vi "Configure Instrument.vi"(0 "RFmx Handle In":refnum<k21>, 1 "Selector String":string, 7 "LO Configuration":T1 {"LO Offset Mode" items=["NoOffset", "Automatic", "User Defined"]; "LO Sharing Mode" items=["None", "Automatic", "Manual"]}, 11 "error in (no error)":errorcluster) -> (4 "RFmx Handle Out":refnum<k21>, 15 "error out":errorcluster)   [LabVIEW 2016, in "RFmxInstr.lvlib"]
uses:
  RFmxInstr.lvlib
  Typedefs/LO Configuration.ctl
  <resource>/objmgr/RFmxInstr.rc
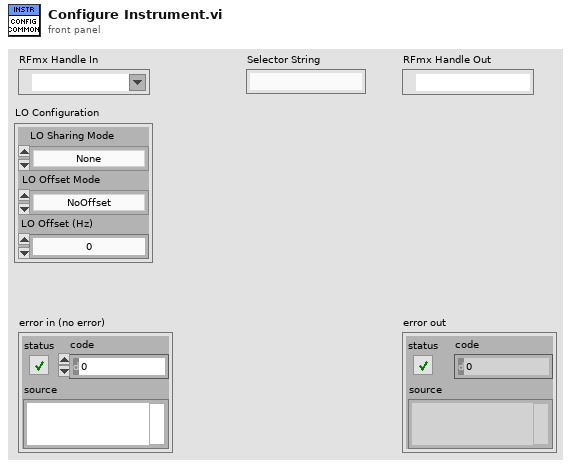
[diagram p1: front panel]
types:
  T1 = typedef "RFmxInstr.lvlib/LO Configuration.ctl" = cluster{"LO Sharing Mode":i32, "LO Offset Mode":i32, "LO Offset (Hz)":dbl}
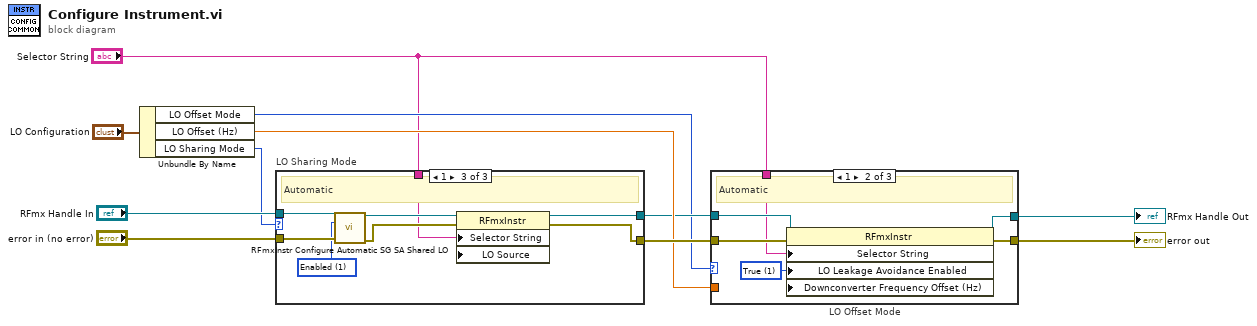
[diagram p0: block diagram]
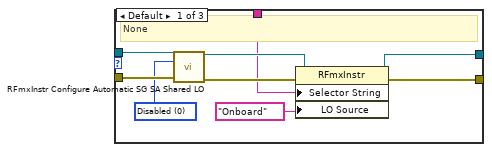
[diagram p2: hidden frame]
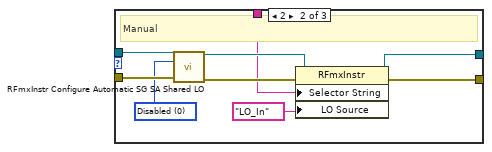
[diagram p3: hidden frame]
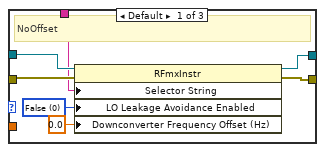
[diagram p4: hidden frame]
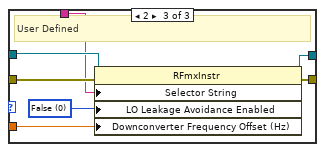
[diagram p5: hidden frame]
diagram:
  n1 = Unbundle By Name("LO Configuration") -> ("LO Offset Mode"=w4:i32, "LO Offset (Hz)"=w8:dbl, "LO Sharing Mode"=w2:i32)
  n2 = case "LO Sharing Mode" shown="1" w2 {
    tunnel: "error in (no error)" -> [w20 w29 w37]
    tunnel: [w16 w25 w33] -> w10
    tunnel: [w15 w24 w32] -> w7
    tunnel: "RFmx Handle In" -> [w19 w28 w36]
    tunnel: "Selector String" -> [w14 w23 w31]
    frame Default {
      w12 = 0 items=["Disabled", "Enabled"] ("Automatic SG SA Shared LO")
      # "None"
      n3 = call <vilib>:"RFmxInstr Configure Automatic SG SA Shared LO.vi"("Instrument Handle In"=w19, "Automatic SG SA Shared LO"=w12, "error in (no error)"=w20) -> ("Instrument Handle Out"=w18:refnum<k21>, "error out"=w17:errorcluster)  [unwired: 11 in]
      n4 = property class="RFmxInstr"(reference=w18, error in=w17, "Selector String"=w14, "LO Source"="Onboard") -> (reference out=w15:refnum<k21>, error out=w16:errorcluster)
    }
    frame 2 {
      w21 = 0 items=["Disabled", "Enabled"] ("Automatic SG SA Shared LO")
      # "Manual"
      n5 = call <vilib>:"RFmxInstr Configure Automatic SG SA Shared LO.vi"("Instrument Handle In"=w28, "Automatic SG SA Shared LO"=w21, "error in (no error)"=w29) -> ("Instrument Handle Out"=w27:refnum<k21>, "error out"=w26:errorcluster)  [unwired: 11 in]
      n6 = property class="RFmxInstr"(reference=w27, error in=w26, "Selector String"=w23, "LO Source"="LO_In") -> (reference out=w24:refnum<k21>, error out=w25:errorcluster)
    }
    frame 1 {
      w30 = 1 items=["Disabled", "Enabled"] ("Automatic SG SA Shared LO")
      # "Automatic"
      n7 = call <vilib>:"RFmxInstr Configure Automatic SG SA Shared LO.vi"("Instrument Handle In"=w36, "Automatic SG SA Shared LO"=w30, "error in (no error)"=w37) -> ("Instrument Handle Out"=w35:refnum<k21>, "error out"=w34:errorcluster)  [unwired: 11 in]
      n8 = property class="RFmxInstr" props=["Selector String", "LO Source"](reference=w35, error in=w34, "Selector String"=w31) -> (reference out=w32:refnum<k21>, error out=w33:errorcluster)  [unwired: 1 in]
    }
  }
  n9 = case "LO Offset Mode" shown="1" w4 {
    tunnel: w10 -> [w43 w50 w55]
    tunnel: [w44 w49 w54] -> w9
    tunnel: w8 -> [_ _ w51]
    tunnel: w7 -> [w42 w48 w57]
    tunnel: [w41 w47 w56] -> w6
    tunnel: "Selector String" -> [w40 w46 w53]
    frame Default {
      w38 = 0 items=["False", "True"] ("LO Leakage Avoidance Enabled")
      # "NoOffset"
      n10 = property class="RFmxInstr"(reference=w42, error in=w43, "Selector String"=w40, "LO Leakage Avoidance Enabled"=w38, "Downconverter Frequency Offset (Hz)"=0.0) -> (reference out=w41:refnum<k21>, error out=w44:errorcluster)
    }
    frame 1 {
      w45 = 1 items=["False", "True"] ("LO Leakage Avoidance Enabled")
      # "Automatic"
      n11 = property class="RFmxInstr" props=["Selector String", "LO Leakage Avoidance Enabled", "Downconverter Frequency Offset (Hz)"](reference=w48, error in=w50, "Selector String"=w46, "LO Leakage Avoidance Enabled"=w45) -> (reference out=w47:refnum<k21>, error out=w49:errorcluster)  [unwired: 1 in]
    }
    frame 2 {
      w52 = 0 items=["False", "True"] ("LO Leakage Avoidance Enabled")
      # "User Defined"
      n12 = property class="RFmxInstr"(reference=w57, error in=w55, "Selector String"=w53, "LO Leakage Avoidance Enabled"=w52, "Downconverter Frequency Offset (Hz)"=w51) -> (reference out=w56:refnum<k21>, error out=w54:errorcluster)
    }
  }
  "error out" <- w9
  "RFmx Handle Out" <- w6
